vi "战舰得分vi.vi"() -> ()   [LabVIEW 2018]
panel:
  out "得分":dbl
  out "战舰爆炸":picture
  out "血量":dbl
  out "战舰血量":T1 scale=0.0..100.0
  out "敌机爆炸":picture
  in  "敌机数量":dbl
  in  "敌机速度":dbl
  out "敌机":picture
  out "按键":dbl
  out "战舰":T2
  out "激光武器1":T3
  out "激光武器 2":T3
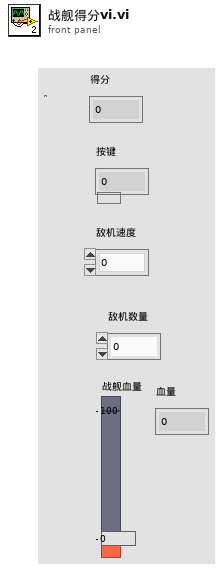
[diagram p1: front panel]
types:
  T1 = typedef "战列巡洋舰_血条.ctl" = dbl
  T2 = typedef "战列巡洋舰.ctl" = picture
  T3 = typedef "战列巡洋舰_激光武器.ctl" = picture
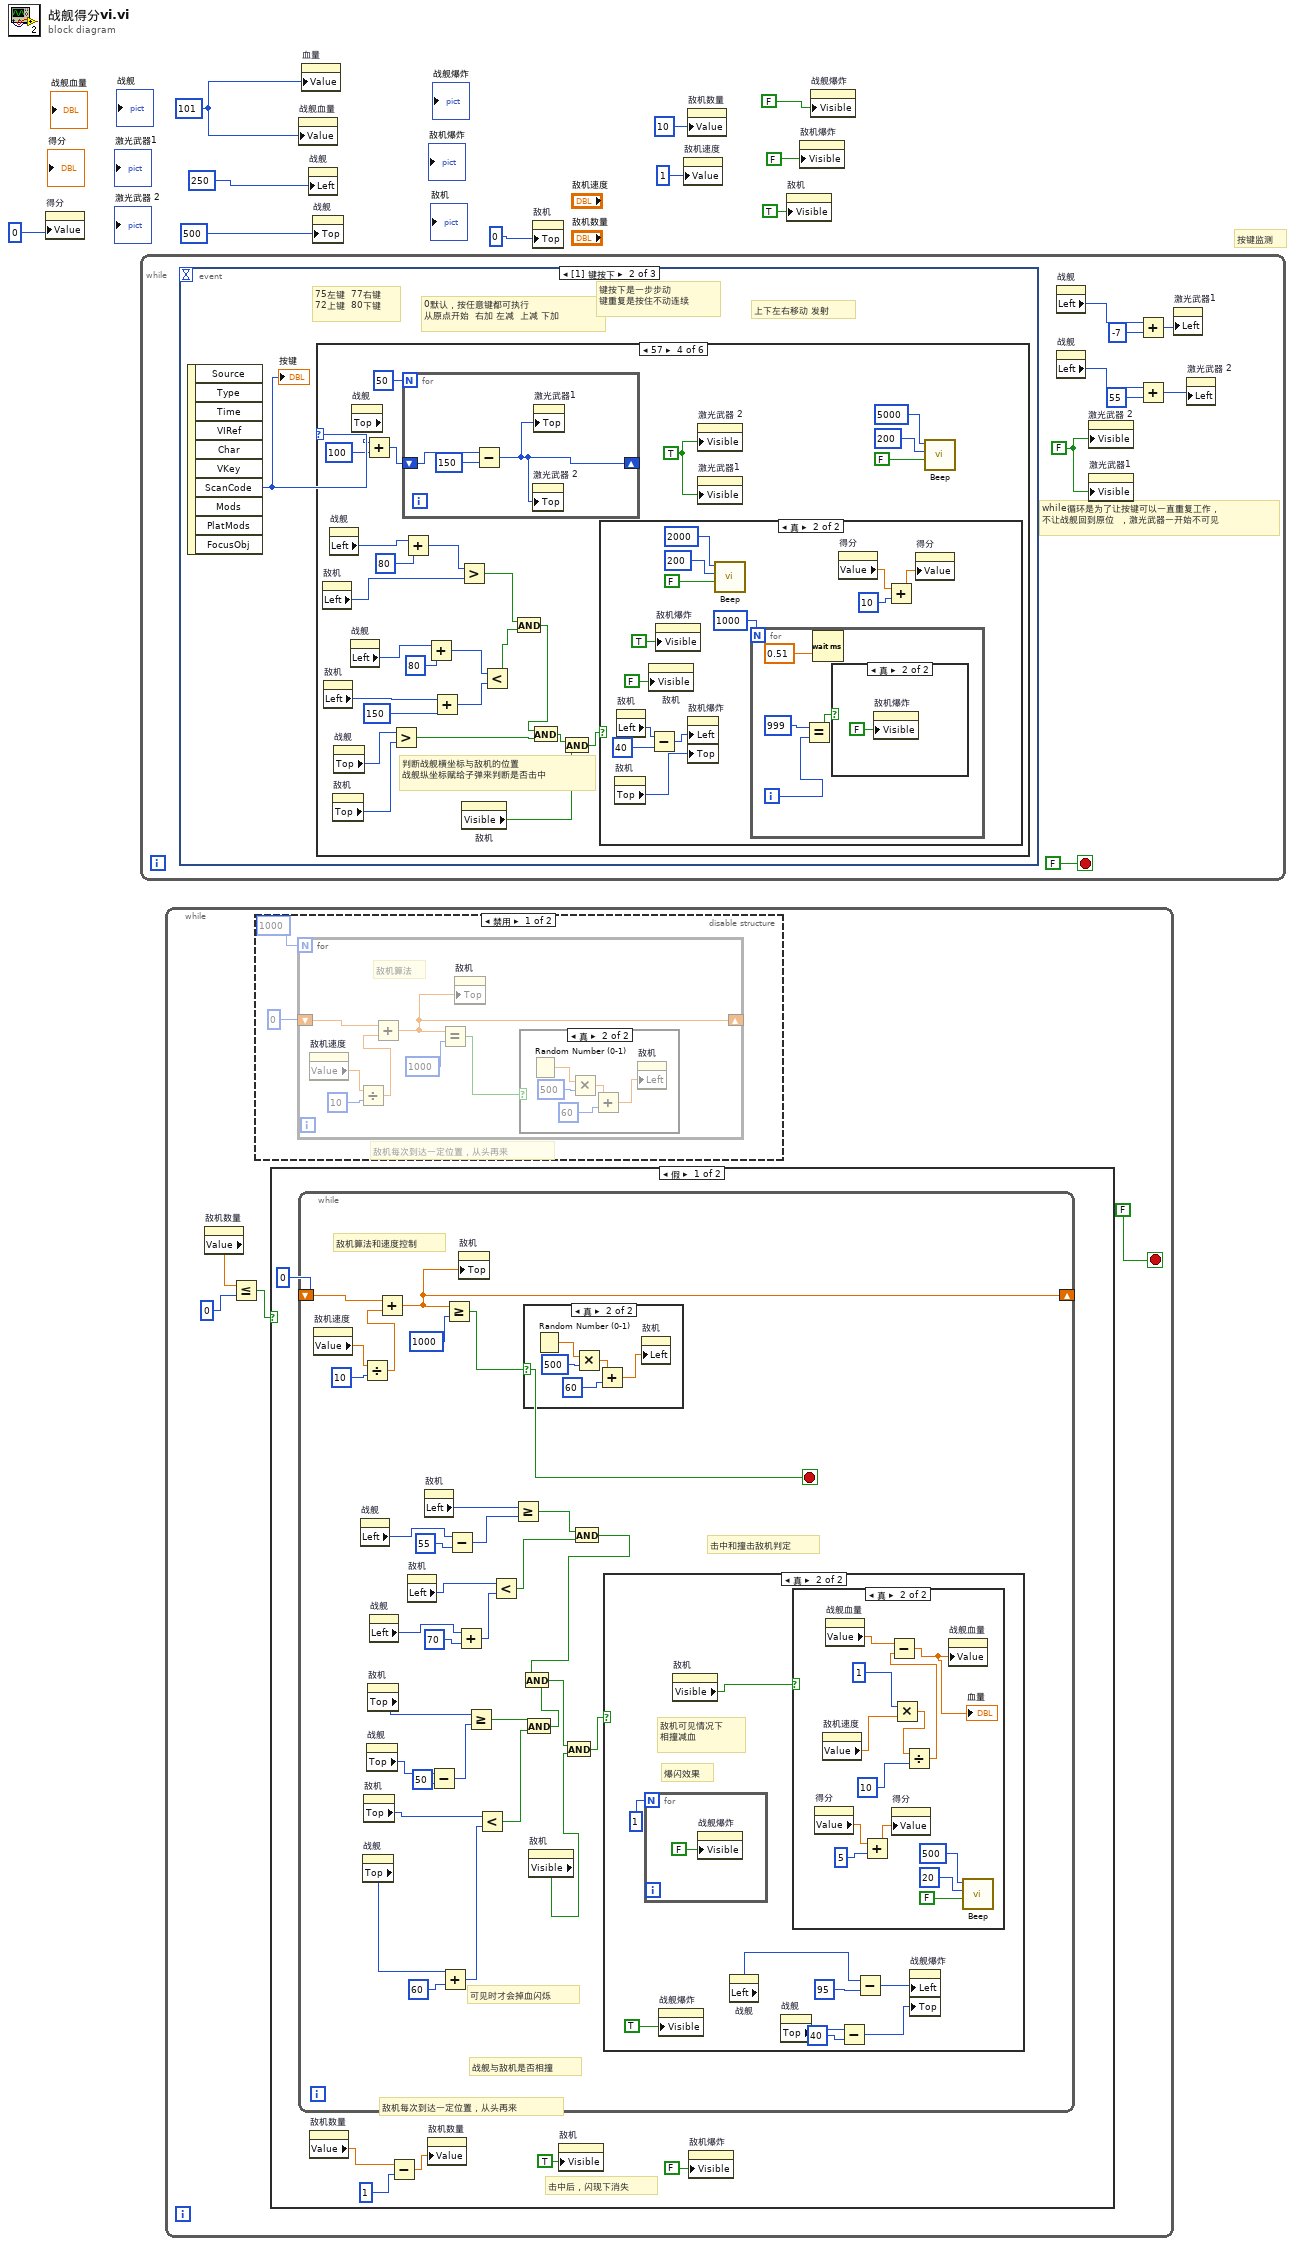
[diagram p0: block diagram]
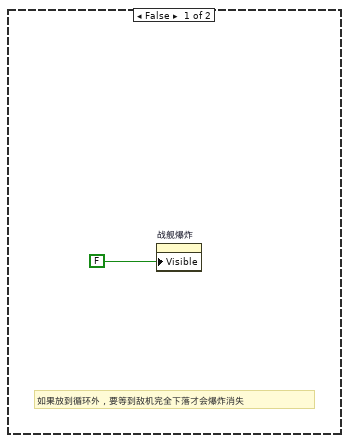
[diagram p2: hidden frame]
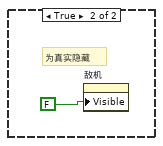
[diagram p5: hidden frame]
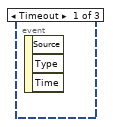
[diagram p8: hidden frame]
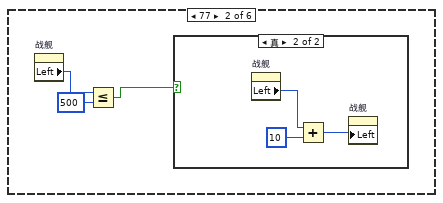
[diagram p10: hidden frame]
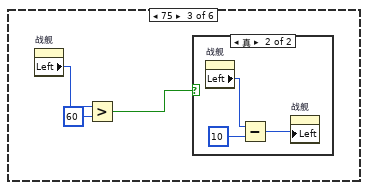
[diagram p12: hidden frame]
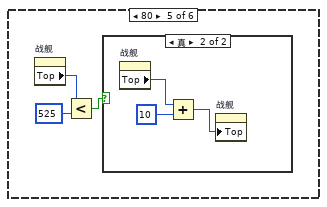
[diagram p16: hidden frame]
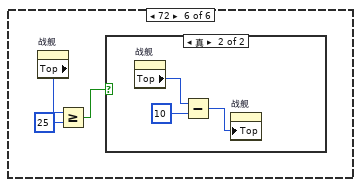
[diagram p18: hidden frame]
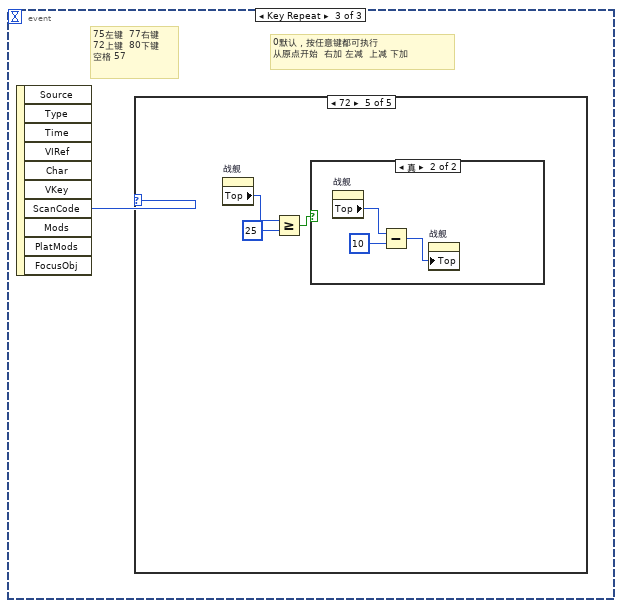
[diagram p20: hidden frame]
diagram:
  w4 = 101
  # "按键监测"
  n1 = property on="得分" class="DigNum (严格)"("Value"=0) -> ()  [unwired: 2 in, 2 out]
  n2 = while {
    stop <- FALSE stop-if-true
    w11 = FALSE
    # "while循环是为了让按键可以一直重复工作，\n不让战舰回到原位  ，激光武器一开始不可见"
    n3 = event shown="[1] 键按下" {
      selector: _ -> [_ _ _]
      dyn-events: _ -> [_ _ _]
      timeout: _ -> [_ _ _]
      event Timeout {
        n4 = event-data() -> ()  [unwired: 1 in, 3 out]
      }
      event Key Down {
        # "上下左右移动 发射"
        # "键按下是一步步动\n键重复是按住不动连续"
        # "75左键  77右键\n72上键  80下键"
        # "0默认，按任意键都可执行\n从原点开始  右加 左减  上减 下加"
        n5 = event-data() -> ("ScanCode"=w19:i16)  [unwired: 1 in, 9 out]
        "按键" <- w19
        n6 = case shown="57" w19 {
          frame 0, Default {
          }
          frame 77 {
            n7 = property on="战舰" class="Pict (严格)"() -> ("Left"=w22:i32)  [unwired: 2 in, 2 out]
            n8 = Less Or Equal?(x=w22, y=500) -> (x <= y?=w20:bool)
            n9 = case shown="真" w20 {
              frame False {
              }
              frame True {
                n10 = property on="战舰" class="Pict (严格)"() -> ("Left"=w24:i32)  [unwired: 2 in, 2 out]
                n11 = Add(x=w24, y=10) -> (x+y=w25:i32)
                n12 = property on="战舰" class="Pict (严格)"("Left"=w25) -> ()  [unwired: 2 in, 2 out]
              }
            }
          }
          frame 75 {
            n13 = property on="战舰" class="Pict (严格)"() -> ("Left"=w28:i32)  [unwired: 2 in, 2 out]
            n14 = Greater?(x=w28, y=60) -> (0:w26:bool)
            n15 = case shown="真" w26 {
              frame False {
              }
              frame True {
                n16 = property on="战舰" class="Pict (严格)"() -> ("Left"=w30:i32)  [unwired: 2 in, 2 out]
                n17 = Subtract(x=w30, y=10) -> (x-y=w31:i32)
                n18 = property on="战舰" class="Pict (严格)"("Left"=w31) -> ()  [unwired: 2 in, 2 out]
              }
            }
          }
          frame 57 {
            w54 = TRUE
            # "判断战舰横坐标与敌机的位置\n战舰纵坐标赋给子弹来判断是否击中"
            n19 = property on="敌机" class="Pict"() -> ("Left"=w51:i32)  [unwired: 2 in, 2 out]
            n20 = property on="敌机" class="Pict"() -> ("Left"=w44:i32)  [unwired: 2 in, 2 out]
            n21 = property on="战舰" class="Pict (严格)"() -> ("Left"=w53:i32)  [unwired: 2 in, 2 out]
            n22 = property on="敌机" class="Pict"() -> ("Top"=w38:i32)  [unwired: 2 in, 2 out]
            n23 = property on="战舰" class="Pict (严格)"() -> ("Top"=w39:i32)  [unwired: 2 in, 2 out]
            n24 = property on="战舰" class="Pict (严格)"() -> ("Left"=w46:i32)  [unwired: 2 in, 2 out]
            n25 = property on="战舰" class="Pict (严格)"() -> ("Top"=w57:i32)  [unwired: 2 in, 2 out]
            n26 = Add(x=w57, y=100) -> (x+y=w55:i32)
            n27 = Greater?(x=w39, y=w38) -> (0:w40:bool)
            n28 = for {
              N: 50 -> [_]
              shift-right: [w77] -> _
              shift-left: w55 -> [w79]
              n29 = Subtract(x=w79, y=150) -> (x-y=w77:i32)
              n30 = property on="激光武器 2" class="Pict (严格)"("Top"=w77) -> ()  [unwired: 2 in, 2 out]
              n31 = property on="激光武器1" class="Pict (严格)"("Top"=w77) -> ()  [unwired: 2 in, 2 out]
            }
            n32 = Add(x=w53, y=80) -> (x+y=w50:i32)
            n33 = Add(x=w46, y=80) -> (x+y=w48:i32)
            n34 = Add(x=w44, y=150) -> (x+y=w43:i32)
            n35 = Greater?(x=w50, y=w51) -> (0:w49:bool)
            n36 = property on="敌机" class="Pict"() -> ("Visible"=w36:bool)  [unwired: 2 in, 2 out]
            n37 = Less?(x=w48, y=w43) -> (x < y?=w45:bool)
            n38 = And(x=w49, y=w45) -> (x .and. y?=w41:bool)
            n39 = And(x=w41, y=w40) -> (x .and. y?=w37:bool)
            n40 = And(x=w37, y=w36) -> (x .and. y?=w35:bool)
            n41 = case shown="真" w35 {
              frame False {
              }
              frame True {
                n42 = property on="敌机" class="Pict"() -> ("Top"=w69:i32)  [unwired: 2 in, 2 out]
                n43 = property on="敌机" class="Pict"() -> ("Left"=w67:i32)  [unwired: 2 in, 2 out]
                n44 = property on="敌机" class="Pict"("Visible"=FALSE ("可见")) -> ()  [unwired: 2 in, 2 out]
                n45 = Subtract(x=w67, y=40) -> (x-y=w66:i32)
                n46 = property on="敌机爆炸" class="Pict"("Visible"=TRUE ("可见")) -> ()  [unwired: 2 in, 2 out]
                n47 = property on="敌机爆炸" class="Pict"("Left"=w66, "Top"=w69) -> ()  [unwired: 2 in, 2 out]
                n48 = call <vilib>:"Beep.vi"("use system alert? (T)"=FALSE, "duration (msec)"=u32 200, "frequency (Hz)"=u32 2000) -> ()  [unwired: 9 in]
                n49 = for {
                  N: 1000 -> [_]
                  i -> [w74]
                  n50 = Equal?(x=999, y=w74) -> (x = y?=w75:bool)
                  n51 = Wait (ms)(milliseconds to wait=0.51) -> ()  [unwired: 1 out]
                  n52 = case shown="真" w75 {
                    frame False {
                    }
                    frame True {
                      n53 = property on="敌机爆炸" class="Pict"("Visible"=FALSE ("可见")) -> ()  [unwired: 2 in, 2 out]
                    }
                  }
                }
                n54 = property on="得分" class="DigNum (严格)"() -> ("Value"=w64:dbl)  [unwired: 2 in, 2 out]
                n55 = Add(x=w64, y=10) -> (x+y=w62:dbl)
                n56 = property on="得分" class="DigNum (严格)"("Value"=w62) -> ()  [unwired: 2 in, 2 out]
              }
            }
            n57 = property on="激光武器 2" class="Pict (严格)"("Visible"=w54) -> ()  [unwired: 2 in, 2 out]
            n58 = property on="激光武器1" class="Pict (严格)"("Visible"=w54) -> ()  [unwired: 2 in, 2 out]
            n59 = call <vilib>:"Beep.vi"("use system alert? (T)"=FALSE, "duration (msec)"=u32 200, "frequency (Hz)"=u32 5000) -> ()  [unwired: 9 in]
          }
          frame 80 {
            n60 = property on="战舰" class="Pict (严格)"() -> ("Top"=w82:i32)  [unwired: 2 in, 2 out]
            n61 = Less?(x=w82, y=525) -> (x < y?=w80:bool)
            n62 = case shown="真" w80 {
              frame False {
              }
              frame True {
                n63 = property on="战舰" class="Pict (严格)"() -> ("Top"=w84:i32)  [unwired: 2 in, 2 out]
                n64 = Add(x=w84, y=10) -> (x+y=w83:i32)
                n65 = property on="战舰" class="Pict (严格)"("Top"=w83) -> ()  [unwired: 2 in, 2 out]
              }
            }
          }
          frame 72 {
            n66 = property on="战舰" class="Pict (严格)"() -> ("Top"=w88:i32)  [unwired: 2 in, 2 out]
            n67 = Greater Or Equal?(x=w88, y=25) -> (x >= y?=w87:bool)
            n68 = case shown="真" w87 {
              frame False {
              }
              frame True {
                n69 = property on="战舰" class="Pict (严格)"() -> ("Top"=w91:i32)  [unwired: 2 in, 2 out]
                n70 = Subtract(x=w91, y=10) -> (x-y=w90:i32)
                n71 = property on="战舰" class="Pict (严格)"("Top"=w90) -> ()  [unwired: 2 in, 2 out]
              }
            }
          }
        }
      }
      event Key Repeat {
        # "75左键  77右键\n72上键  80下键\n空格 57"
        # "0默认，按任意键都可执行\n从原点开始  右加 左减  上减 下加"
        n72 = event-data() -> ("ScanCode"=w92:i16)  [unwired: 1 in, 9 out]
        n73 = case shown="72" w92 {
          frame 0, Default {
          }
          frame 77 {
            n74 = property on="战舰" class="Pict (严格)"() -> ("Left"=w95:i32)  [unwired: 2 in, 2 out]
            n75 = Less Or Equal?(x=w95, y=500) -> (x <= y?=w94:bool)
            n76 = case shown="真" w94 {
              frame False {
              }
              frame True {
                n77 = property on="战舰" class="Pict (严格)"() -> ("Left"=w97:i32)  [unwired: 2 in, 2 out]
                n78 = Add(x=w97, y=10) -> (x+y=w98:i32)
                n79 = property on="战舰" class="Pict (严格)"("Left"=w98) -> ()  [unwired: 2 in, 2 out]
              }
            }
          }
          frame 75 {
            n80 = property on="战舰" class="Pict (严格)"() -> ("Left"=w101:i32)  [unwired: 2 in, 2 out]
            n81 = Greater Or Equal?(x=w101, y=25) -> (x >= y?=w100:bool)
            n82 = case shown="真" w100 {
              frame False {
              }
              frame True {
                n83 = property on="战舰" class="Pict (严格)"() -> ("Left"=w104:i32)  [unwired: 2 in, 2 out]
                n84 = Subtract(x=w104, y=10) -> (x-y=w103:i32)
                n85 = property on="战舰" class="Pict (严格)"("Left"=w103) -> ()  [unwired: 2 in, 2 out]
              }
            }
          }
          frame 80 {
            n86 = property on="战舰" class="Pict (严格)"() -> ("Top"=w107:i32)  [unwired: 2 in, 2 out]
            n87 = Less Or Equal?(x=w107, y=525) -> (x <= y?=w106:bool)
            n88 = case shown="真" w106 {
              frame False {
              }
              frame True {
                n89 = property on="战舰" class="Pict (严格)"() -> ("Top"=w109:i32)  [unwired: 2 in, 2 out]
                n90 = Add(x=w109, y=10) -> (x+y=w108:i32)
                n91 = property on="战舰" class="Pict (严格)"("Top"=w108) -> ()  [unwired: 2 in, 2 out]
              }
            }
          }
          frame 72 {
            n92 = property on="战舰" class="Pict (严格)"() -> ("Top"=w113:i32)  [unwired: 2 in, 2 out]
            n93 = Greater Or Equal?(x=w113, y=25) -> (x >= y?=w112:bool)
            n94 = case shown="真" w112 {
              frame False {
              }
              frame True {
                n95 = property on="战舰" class="Pict (严格)"() -> ("Top"=w116:i32)  [unwired: 2 in, 2 out]
                n96 = Subtract(x=w116, y=10) -> (x-y=w115:i32)
                n97 = property on="战舰" class="Pict (严格)"("Top"=w115) -> ()  [unwired: 2 in, 2 out]
              }
            }
          }
        }
      }
    }
    n98 = property on="战舰" class="Pict (严格)"() -> ("Left"=w17:i32)  [unwired: 2 in, 2 out]
    n99 = property on="战舰" class="Pict (严格)"() -> ("Left"=w13:i32)  [unwired: 2 in, 2 out]
    n100 = property on="激光武器 2" class="Pict (严格)"("Visible"=w11) -> ()  [unwired: 2 in, 2 out]
    n101 = property on="激光武器1" class="Pict (严格)"("Visible"=w11) -> ()  [unwired: 2 in, 2 out]
    n102 = Add(x=w17, y=-7) -> (x+y=w16:i32)
    n103 = Add(x=w13, y=55) -> (x+y=w12:i32)
    n104 = property on="激光武器1" class="Pict (严格)"("Left"=w16) -> ()  [unwired: 2 in, 2 out]
    n105 = property on="激光武器 2" class="Pict (严格)"("Left"=w12) -> ()  [unwired: 2 in, 2 out]
  }
  n106 = while {
    stop <- FALSE stop-if-true
    n107 = property on="敌机数量" class="DigNum (严格)"() -> ("Value"=w119:dbl)  [unwired: 2 in, 2 out]
    n108 = Less Or Equal?(x=w119, y=0) -> (x <= y?=w117:bool)
    n109 = disable-structure shown="禁用" {
      frame Disabled {
        # "敌机每次到达一定位置，从头再来"
        n110 = for {
          N: 1000 -> [_]
          shift-right: [w194] -> _
          shift-left: 0 -> [w197]
          # "敌机算法"
          n111 = property on="敌机速度" class="DigNum (严格)"() -> ("Value"=w193:dbl)  [unwired: 2 in, 2 out]
          n112 = Divide(x=w193, y=10) -> (x/y=w192:dbl)
          n113 = Add(x=w197, y=w192) -> (x+y=w194:dbl)
          n114 = Equal?(x=w194, y=1000) -> (x = y?=w195:bool)
          n115 = property on="敌机" class="Pict"("Top"=w194) -> ()  [unwired: 2 in, 2 out]
          n116 = case shown="真" w195 {
            frame False {
            }
            frame True {
              n117 = Random Number (0-1)() -> (number: 0 to 1=w202:dbl)
              n118 = Multiply(x=w202, y=500) -> (x*y=w200:dbl)
              n119 = Add(x=w200, y=60) -> (x+y=w199:dbl)
              n120 = property on="敌机" class="Pict"("Left"=w199) -> ()  [unwired: 2 in, 2 out]
            }
          }
        }
      }
      frame Enabled {
      }
    }
    n121 = case shown="假" w117 {
      frame False {
        # "击中后，闪现下消失"
        # "敌机每次到达一定位置，从头再来"
        n122 = while {
          shift-right: [w156] -> _
          shift-left: 0 -> [w158]
          stop <- w152 stop-if-true
          # "击中和撞击敌机判定"
          # "可见时才会掉血闪烁"
          # "战舰与敌机是否相撞"
          # "敌机算法和速度控制"
          n123 = property on="敌机速度" class="DigNum (严格)"() -> ("Value"=w155:dbl)  [unwired: 2 in, 2 out]
          n124 = property on="战舰" class="Pict (严格)"() -> ("Left"=w150:i32)  [unwired: 2 in, 2 out]
          n125 = Divide(x=w155, y=10) -> (x/y=w154:dbl)
          n126 = property on="战舰" class="Pict (严格)"() -> ("Top"=w134:i32)  [unwired: 2 in, 2 out]
          n127 = property on="敌机" class="Pict"() -> ("Top"=w133:i32)  [unwired: 2 in, 2 out]
          n128 = property on="战舰" class="Pict (严格)"() -> ("Top"=w140:i32)  [unwired: 2 in, 2 out]
          n129 = property on="敌机" class="Pict"() -> ("Top"=w141:i32)  [unwired: 2 in, 2 out]
          n130 = property on="战舰" class="Pict (严格)"() -> ("Left"=w144:i32)  [unwired: 2 in, 2 out]
          n131 = Add(x=w158, y=w154) -> (x+y=w156:dbl)
          n132 = property on="敌机" class="Pict"() -> ("Left"=w146:i32)  [unwired: 2 in, 2 out]
          n133 = property on="敌机" class="Pict"() -> ("Left"=w151:i32)  [unwired: 2 in, 2 out]
          n134 = Subtract(x=w140, y=50) -> (x-y=w138:i32)
          n135 = Add(x=w134, y=60) -> (x+y=w136:i32)
          n136 = Greater Or Equal?(x=w156, y=1000) -> (x >= y?=w152:bool)
          n137 = Subtract(x=w150, y=55) -> (x-y=w149:i32)
          n138 = Add(x=w144, y=70) -> (x+y=w143:i32)
          n139 = property on="敌机" class="Pict"("Top"=w156) -> ()  [unwired: 2 in, 2 out]
          n140 = Greater Or Equal?(x=w141, y=w138) -> (x >= y?=w132:bool)
          n141 = Less?(x=w133, y=w136) -> (x < y?=w131:bool)
          n142 = Less?(x=w146, y=w143) -> (x < y?=w142:bool)
          n143 = Greater Or Equal?(x=w151, y=w149) -> (x >= y?=w147:bool)
          n144 = case shown="真" w152 {
            frame False {
            }
            frame True {
              n145 = Random Number (0-1)() -> (number: 0 to 1=w187:dbl)
              n146 = Multiply(x=w187, y=500) -> (x*y=w185:dbl)
              n147 = Add(x=w185, y=60) -> (x+y=w184:dbl)
              n148 = property on="敌机" class="Pict"("Left"=w184) -> ()  [unwired: 2 in, 2 out]
            }
          }
          n149 = And(x=w132, y=w131) -> (x .and. y?=w130:bool)
          n150 = property on="敌机" class="Pict"() -> ("Visible"=w128:bool)  [unwired: 2 in, 2 out]
          n151 = And(x=w147, y=w142) -> (x .and. y?=w137:bool)
          n152 = And(x=w137, y=w130) -> (x .and. y?=w129:bool)
          n153 = And(x=w129, y=w128) -> (x .and. y?=w127:bool)
          n154 = case shown="真" w127 {
            frame False {
              # "如果放到循环外，要等到敌机完全下落才会爆炸消失"
              n155 = property on="战舰爆炸" class="Pict"("Visible"=FALSE ("可见")) -> ()  [unwired: 2 in, 2 out]
            }
            frame True {
              # "爆闪效果"
              # "敌机可见情况下\n相撞减血"
              n156 = for {
                N: 1 -> [_]
                n157 = property on="战舰爆炸" class="Pict"("Visible"=FALSE ("可见")) -> ()  [unwired: 2 in, 2 out]
              }
              n158 = property on="战舰爆炸" class="Pict"("Visible"=TRUE ("可见")) -> ()  [unwired: 2 in, 2 out]
              n159 = property on="敌机" class="Pict"() -> ("Visible"=w168:bool)  [unwired: 2 in, 2 out]
              n160 = property on="战舰" class="Pict (严格)"() -> ("Left"=w166:i32)  [unwired: 2 in, 2 out]
              n161 = property on="战舰" class="Pict (严格)"() -> ("Top"=w163:i32)  [unwired: 2 in, 2 out]
              n162 = case shown="真" w168 {
                frame False {
                }
                frame True {
                  n163 = property on="得分" class="DigNum (严格)"() -> ("Value"=w175:dbl)  [unwired: 2 in, 2 out]
                  n164 = property on="敌机速度" class="DigNum (严格)"() -> ("Value"=w181:dbl)  [unwired: 2 in, 2 out]
                  n165 = property on="战舰血量" class="Slide (严格)"() -> ("Value"=w182:T1)  [unwired: 2 in, 2 out]
                  n166 = Add(x=w175, y=5) -> (x+y=w174:dbl)
                  n167 = Multiply(x=1, y=w181) -> (x*y=w180:dbl)
                  n168 = property on="得分" class="DigNum (严格)"("Value"=w174) -> ()  [unwired: 2 in, 2 out]
                  n169 = Divide(x=w180, y=10) -> (x/y=w177:dbl)
                  n170 = Subtract(x=w182, y=w177) -> (x-y=w176:T1)
                  "血量" <- w176
                  n171 = property on="战舰血量" class="Slide (严格)"("Value"=w176) -> ()  [unwired: 2 in, 2 out]
                  n172 = call <vilib>:"Beep.vi"("use system alert? (T)"=FALSE, "duration (msec)"=u32 20, "frequency (Hz)"=u32 500) -> ()  [unwired: 9 in]
                }
              }
              n173 = Subtract(x=w163, y=40) -> (x-y=w161:i32)
              n174 = Subtract(x=w166, y=95) -> (x-y=w164:i32)
              n175 = property on="战舰爆炸" class="Pict"("Left"=w164, "Top"=w161) -> ()  [unwired: 2 in, 2 out]
            }
          }
        }
        n176 = property on="敌机数量" class="DigNum (严格)"() -> ("Value"=w124:dbl)  [unwired: 2 in, 2 out]
        n177 = Subtract(x=w124, y=1) -> (x-y=w125:dbl)
        n178 = property on="敌机数量" class="DigNum (严格)"("Value"=w125) -> ()  [unwired: 2 in, 2 out]
        n179 = property on="敌机" class="Pict"("Visible"=TRUE ("可见")) -> ()  [unwired: 2 in, 2 out]
        n180 = property on="敌机爆炸" class="Pict"("Visible"=FALSE ("可见")) -> ()  [unwired: 2 in, 2 out]
      }
      frame True {
        # "为真实隐藏"
        n181 = property on="敌机" class="Pict"("Visible"=FALSE ("可见")) -> ()  [unwired: 2 in, 2 out]
      }
    }
  }
  n182 = property on="战舰血量" class="Slide (严格)"("Value"=w4) -> ()  [unwired: 2 in, 2 out]
  n183 = property on="血量" class="DigNum (严格)"("Value"=w4) -> ()  [unwired: 2 in, 2 out]
  n184 = property on="战舰" class="Pict (严格)"("Left"=250 ("位置:居左")) -> ()  [unwired: 2 in, 2 out]
  n185 = property on="战舰" class="Pict (严格)"("Top"=500 ("位置:置顶")) -> ()  [unwired: 2 in, 2 out]
  n186 = property on="敌机" class="Pict"("Top"=0) -> ()  [unwired: 2 in, 2 out]
  n187 = property on="敌机速度" class="DigNum (严格)"("Value"=1) -> ()  [unwired: 2 in, 2 out]
  n188 = property on="敌机数量" class="DigNum (严格)"("Value"=10) -> ()  [unwired: 2 in, 2 out]
  n189 = property on="敌机" class="Pict"("Visible"=TRUE ("可见")) -> ()  [unwired: 2 in, 2 out]
  n190 = property on="敌机爆炸" class="Pict"("Visible"=FALSE ("可见")) -> ()  [unwired: 2 in, 2 out]
  n191 = property on="战舰爆炸" class="Pict"("Visible"=FALSE ("可见")) -> ()  [unwired: 2 in, 2 out]
